vi "1WIRE_ReadBit.vi"(8 "error in":errorcluster) -> (0 "error out":errorcluster, 2 "Bit Read":bool)   [LabVIEW 2013]
doc: "This VI is created by Vincent Claes for FPDA-1 more information on http://pwo.fpga.be\n\nvincent.claes@xios.be\nclaesvincent@gmail.com\n\nhttp://www.linkedin.com/in/vincentclaes"
uses:
  <vilib>/eio/EIONode/EIONode.xnode
  <vilib>/eio/EIOMethodNode/EIOMethodNode.xnode
  <vilib>/rvi/eio/common/nirviEmuTemplateMethod_errors.vi
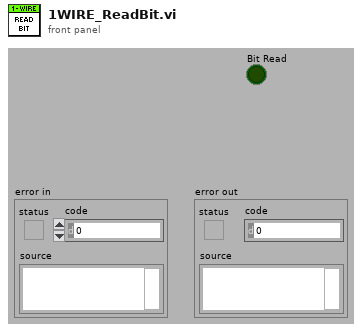
[diagram p1: front panel]
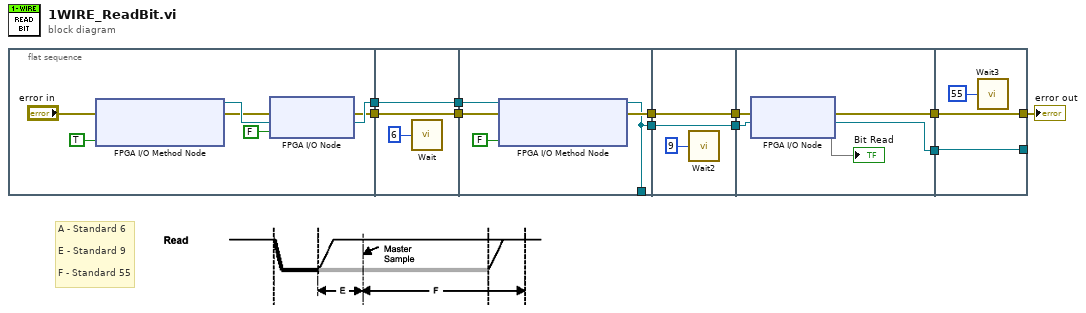
[diagram p0: block diagram]
diagram:
  # "A - Standard 6\n\nE - Standard 9\n\nF - Standard 55"
  n1 = flat-sequence {
    tunnel: [w16] -> w11
    tunnel: [w15] -> w5
    tunnel: w11 -> [w20]
    tunnel: [w20] -> w10
    tunnel: w5 -> [w19]
    tunnel: [w19] -> w4
    tunnel: w10 -> [w26]
    tunnel: [w23] -> w8
    tunnel: [w25] -> w6
    tunnel: w4 -> [w24]
    tunnel: [w23] -> _
    tunnel: [w28] -> w9
    tunnel: w8 -> [w28]
    tunnel: [w27] -> w7
    tunnel: w6 -> [w27]
    tunnel: w9 -> [w33]
    tunnel: w7 -> [w32]
    tunnel: [w31] -> w3
    tunnel: [w30] -> w1
    tunnel: [w36] -> w2
    tunnel: w3 -> [w36]
    tunnel: [w35] -> _
    tunnel: w1 -> [w35]
    frame #0 {
      n2 = xnode "FPGA I/O Method Node"("error in"="error in", "Enable"=TRUE) -> ("error out"=w14:errorcluster, "FPGA I/O Out"=w17:refnum<k21>)  [unwired: 1 in]
      n3 = xnode "FPGA I/O Node"("error in"=w14, "I/O Item"=FALSE ("FX2_IO1_J1_0"), "FPGA I/O In"=w17) -> ("error out"=w15:errorcluster, "FPGA I/O Out"=w16:refnum<k21>)
    }
    frame #1 {
      n4 = call "Wait"("Count(uSec)"=u32 6) -> ()  [unwired: 1 out]
    }
    frame #2 {
      n5 = xnode "FPGA I/O Method Node"("error in"=w24, "FPGA I/O In"=w26, "Enable"=FALSE) -> ("error out"=w25:errorcluster, "FPGA I/O Out"=w23:refnum<k21>)
    }
    frame #3 {
      n6 = call "Wait2"("Count(uSec)"=u32 9) -> ()  [unwired: 1 out]
    }
    frame #4 {
      n7 = xnode "FPGA I/O Node"("error in"=w32, "FPGA I/O In"=w33) -> ("error out"=w31:errorcluster, "I/O Item"=→"Bit Read", "FPGA I/O Out"=w30:refnum<k21>)
    }
    frame #5 {
      n8 = call "Wait3"("Count(uSec)"=u32 55) -> ()  [unwired: 1 out]
    }
  }
  "error out" <- w2
